vi "UDPReceiver.vi"(8 "error in (no error)":errorcluster, 11 "ImageStreamViewer in":refnum<class "ImageStreamViewer.lvclass">) -> (0 "error out":errorcluster, 3 "ImageStreamViewer out":refnum<class "ImageStreamViewer.lvclass">)   [LabVIEW 2011, in "Views.lvlib" / "Camera.lvlib" / "ImageStreamViewer.lvclass"]
uses:
  ImageStreamViewer.lvclass
panel:
  in  "Port":u16=61557
  in  "reset":bool
  in  "stop":bool
  out "Data Received":string
  in  "max bytes/read":i32=548
  out "# of Bytes Received":i32
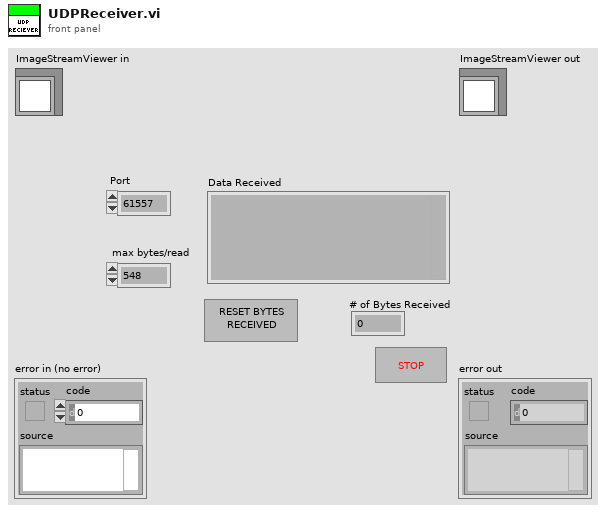
[diagram p1: front panel]
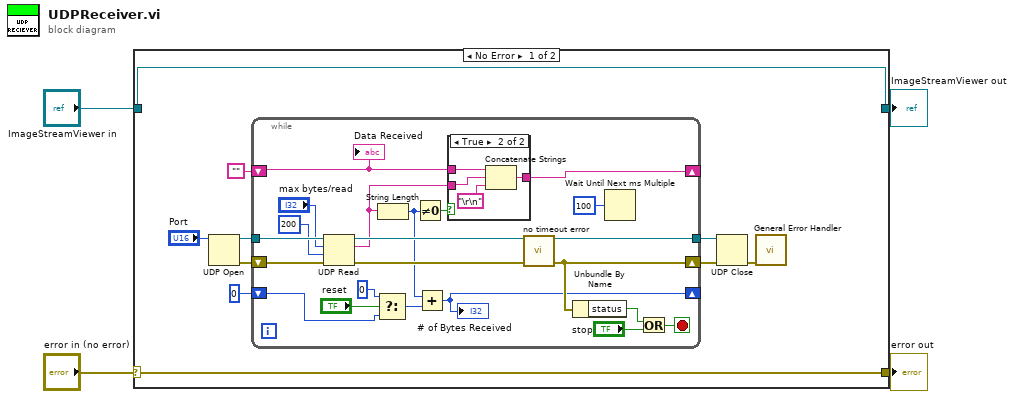
[diagram p0: block diagram]
diagram:
  n1 = case shown="No Error" "error in (no error)" {
    selector: "error in (no error)" -> [w13 w42]
    tunnel: [w13 w42] -> w3
    tunnel: [w14 w41] -> w1
    tunnel: "ImageStreamViewer in" -> [w14 w41]
    frame No Error {
      n2 = UDP Open(11:"Port") -> (port=w7:refnum<k16>, 0:w6:errorcluster)  [unwired: 4 in, 1 out]
      n3 = while {
        shift-left: "" -> [w18]
        shift-right: [w17] -> _
        shift-left: 0 -> [w23]
        shift-right: [w25] -> _
        tunnel: [w33] -> w8
        tunnel: w7 -> [w34]
        shift-left: w6 -> [w35]
        shift-right: [w27] -> w9
        stop <- w30 stop-if-true
        n4 = UDP Read(connection ID=w34, max size (548)="max bytes/read", timeout ms (25000)=200, 8:w35) -> (data out=w19:string, error out=w28:errorcluster, 3:w33:refnum<k16>)  [unwired: 2 out]
        n5 = Select(t=0, s="reset", f=w23) -> (s? t:f=w22:i32)
        n6 = String Length(string=w19) -> (length=w16:i32)
        n7 = Not Equal To 0?(x=w16) -> (x != 0?=w15:bool)
        n8 = Add(x=w16, y=w22) -> (x+y=w25:i32)
        "# of Bytes Received" <- w25
        n9 = case shown="True" w15 {
          tunnel: w18 -> [w36 w40]
          tunnel: w19 -> [_ w38]
          tunnel: [w36 w39] -> w17
          frame False {
          }
          frame True {
            n10 = Concatenate Strings(w40, w38, "\r\n" ("Substring")) -> (w39:string)
          }
        }
        n11 = call "no timeout error.vi"("error in (no error)"=w28) -> ("error out"=w27:errorcluster)
        n12 = Unbundle By Name(w27) -> ("status"=w29:bool)
        n13 = Wait Until Next ms Multiple(millisecond multiple=u32 100) -> ()  [unwired: 1 out]
        n14 = Or(x=w29, y="stop") -> (x .or. y?=w30:bool)
        "Data Received" <- w18
      }
      n15 = UDP Close(connection ID=w8, 8:w9) -> (error out=w10:errorcluster)  [unwired: 1 out]
      n16 = call <vilib>:"General Error Handler.vi"("error in (no error)"=w10) -> ()  [unwired: 10 in, 5 out]
    }
    frame Error {
    }
  }
  "error out" <- w3
  "ImageStreamViewer out" <- w1
